vi "myRIO_BRig_RT_dataLick_LeftRightBoth.vi"() -> (2 "output_LeftRightBoth":i32)   [LabVIEW 2014]
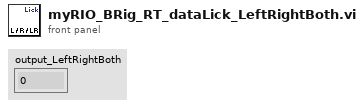
[diagram p1: front panel]
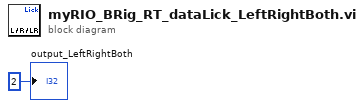
[diagram p0: block diagram]
diagram:
  "output_LeftRightBoth" <- 2 ("output_iBlock")
